vi "Read Application Settings.vi"(8 "error in (no error)":errorcluster, 11 "Application in":refnum<class "Application.lvclass">) -> (0 "error out":errorcluster, 2 "ApplicationSettings":T1, 3 "Application out":refnum<class "Application.lvclass">)   [LabVIEW 2019, in "Application.lvclass"]
uses:
  Application.lvclass
  ApplicationSettings.ctl
  RobotType.ctl
  Application.lvclass/Application.ctl
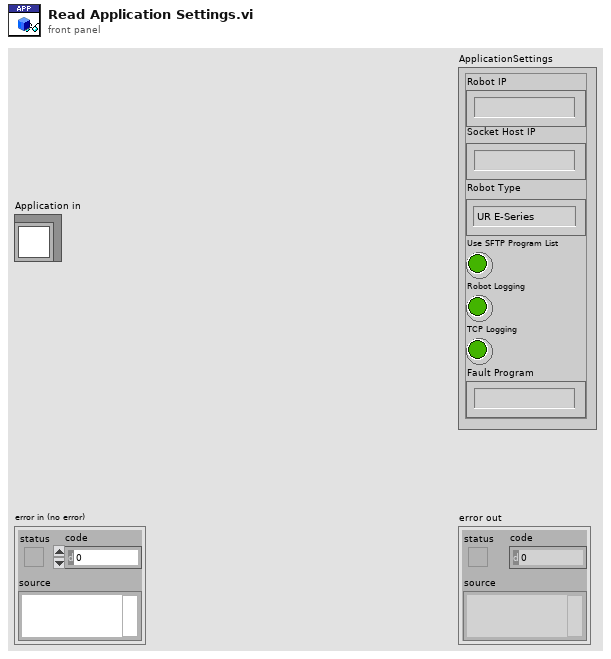
[diagram p1: front panel]
types:
  T1 = typedef "Application.lvclass/ApplicationSettings.ctl" = cluster{"Robot IP":string, "Socket Host IP":string, "Robot Type":T2, "Use SFTP Program List":bool, "Robot Logging":bool, "TCP Logging":bool, "Fault Program":string}
  T2 = typedef "Application.lvclass/RobotType.ctl" = enum16{"UR E-Series", "UR CB-Series"}
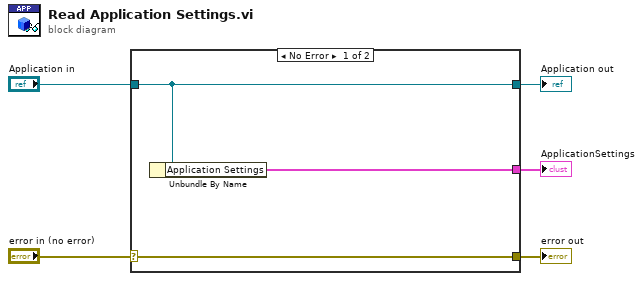
[diagram p0: block diagram]
diagram:
  n1 = case shown="No Error" "error in (no error)" {
    selector: "error in (no error)" -> [w8 w9]
    tunnel: [w8 w9] -> w4
    tunnel: [w7 w10] -> w2
    tunnel: "Application in" -> [w7 w10]
    tunnel: [w6 _] -> w1
    frame No Error {
      n2 = Unbundle By Name(w7) -> ("Application Settings"=w6:T1)
    }
    frame Error {
    }
  }
  "error out" <- w4
  "Application out" <- w2
  "ApplicationSettings" <- w1
